vi "check actions output.vi"(8 "error in":errorcluster, 11 "Actions IN":T1) -> (0 "error in 2":errorcluster)   [LabVIEW 2016]
panel:
  out "Actions OUT":T1
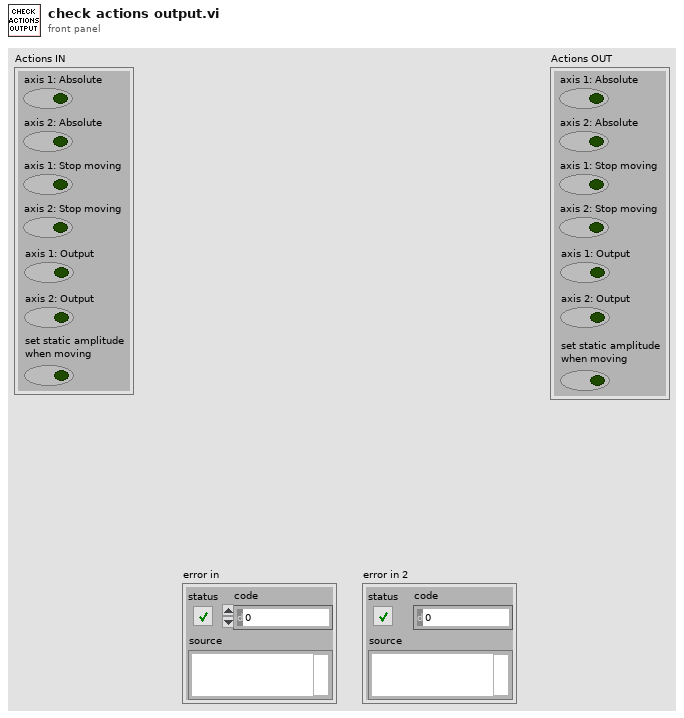
[diagram p1: front panel]
types:
  T1 = cluster{"axis 1: Absolute":bool, "axis 2: Absolute":bool, "axis 1: Stop moving":bool, "axis 2: Stop moving":bool, "axis 1: Output":bool, "axis 2: Output":bool, "set static amplitude\nwhen moving":bool}
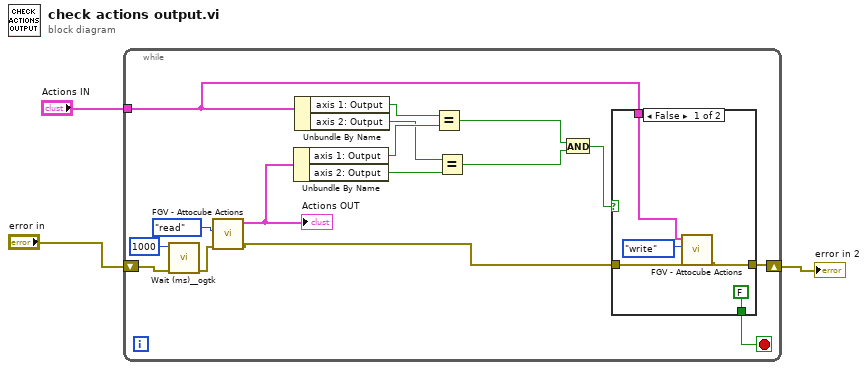
[diagram p0: block diagram]
diagram:
  n1 = while {
    shift-right: [w17] -> w2
    shift-left: "error in" -> [w6]
    tunnel: "Actions IN" -> [w7]
    stop <- w18 stop-if-true
    n2 = call <userlib>:"Wait (ms)__ogtk.vi"("error in (no error)"=w6, "milliseconds to wait"=u32 1000) -> ("error out"=w5:errorcluster)  [unwired: 8 in, 1 out]
    n3 = call "FGV - Attocube Actions.vi"("error in"=w5, "Function"=enum16{"write", "read"}."read") -> ("error out"=w16:errorcluster, "Actions OUT"=w14:T1)  [unwired: 4 in]
    "Actions OUT" <- w14
    n4 = Unbundle By Name(w14) -> ("axis 1: Output"=w12:bool, "axis 2: Output"=w10:bool)
    n5 = Unbundle By Name(w7) -> ("axis 1: Output"=w13:bool, "axis 2: Output"=w11:bool)
    n6 = Equal?(x=w13, y=w12) -> (x = y?=w9:bool)
    n7 = Equal?(x=w11, y=w10) -> (x = y?=w8:bool)
    n8 = And(x=w9, y=w8) -> (x .and. y?=w19:bool)
    n9 = case shown="False" w19 {
      selector: w19 -> [_ w26]
      tunnel: [FALSE w26] -> w18
      tunnel: w16 -> [w22 w25]
      tunnel: [w21 w25] -> w17
      tunnel: w7 -> [w20 _]
      frame False {
        n10 = call "FGV - Attocube Actions.vi"("error in"=w22, "Function"=enum16{"write", "read"}."write", "Actions IN"=w20) -> ("error out"=w21:errorcluster)  [unwired: 3 in, 1 out]
      }
      frame True {
      }
    }
  }
  "error in 2" <- w2
